vi "Main.vi"(11 "Module Admin":refnum<class "Delacor_lib_QMH_Module Admin.lvclass">) -> ()   [LabVIEW 2023, in "DeviceManager.lvlib"]
doc: "This template is based off of the Queued Message Handler design pattern and the Queued Message Handler project template that ships with LabVIEW.\n\nThe main difference is that the queue is private to this module and communication between modules is performed via Broadcast and Request events.\n\nRequest events are wrapped in public API methods and are handled in the Event Handling Loop (EHL) of this VI. Any module can register for Broadcast events sent by this module. The EHL generates messages based on user interface actions.\n\nThe Message Handling Loop (MHL) processes messages generated by the EHL, or by other messages. The messages are string values, so new messages can be added easily to the Message Cases case structure in the MHL. Each message cluster can also provide an optional value for Message Data, which is a variant that can be converted to whatever message-specific data is required.\n_____\nBased on DQMH Project Template 7.0.0.1280."
uses:
  DeviceManager.lvlib
  <vilib>/Delacor/Delacor QMH/Libraries/Module Admin_class/Delacor_lib_QMH_Module Admin.lvclass
  Module Data--cluster.ctl
  ICLcommuncationData.ctl
  Classes/Communicator/Communicator.lvclass
  OpenWebSocketCommunication (Reply Payload)--cluster.ctl
  SendJSONandAskForReply (Reply Payload)--cluster.ctl
  DiscoverDevices (Reply Payload)--cluster.ctl
  Classes/Mono/Monochromator.lvclass
  Classes/CCD/CCD.lvclass
  Classes/SCD/SCD.lvclass
  <vilib>/Delacor/Delacor QMH/Libraries/Message Queue_class/Delacor_lib_QMH_Message Queue.lvclass/Delacor_lib_QMH_Message Queue.ctl
  Stop Argument--cluster.ctl
  <vilib>/Delacor/Delacor QMH/Libraries/Module Admin_class/Delacor_lib_QMH_Module Admin.lvclass/Delacor_lib_QMH_Module Admin.ctl
  <vilib>/Utility/miscctls.llb/LVPointTypeDef.ctl
  <vilib>/Delacor/Delacor QMH/Libraries/Message Queue_class/Delacor_lib_QMH_Enqueue Message (Single).vi
  <vilib>/Delacor/Delacor QMH/Libraries/Module Admin_class/Delacor_lib_QMH_Get External Launch.vi
  522d4d4e-e2b9-4a0b-813b-57f0bcdbaa64.vi
  <vilib>/GPower/Error/Library/ErrorType.vi
  <vilib>/GPower/Error/Library/SplitAppended.vi
  <vilib>/Utility/error.llb/Trim Whitespace.vi
  <vilib>/GPower/Error/Library/SubVIs/ExplanationToError.vi
  <vilib>/Utility/error.llb/Trim Whitespace One-Sided.vi
  <vilib>/dlg_ctls.llb/Space Constant.vi
  <vilib>/Utility/error.llb/Error Code Database.vi
  <vilib>/GPower/Error/Library/SubVIs/SetStatus.vi
  <vilib>/GPower/Error/Library/AppendErrors.vi
  <vilib>/GPower/Error/Library/Append/AppendSingle.vi
  <vilib>/Delacor/Delacor QMH/Libraries/Message Queue_class/Delacor_lib_QMH_Message Queue.lvclass
  <vilib>/JKI/JKI DotNet System Exec/dotnet_system_exec/dotnet_system_exec.lvclass
  <vilib>/GPower/Error/GPError.lvlib
panel:
  out "ICL output":string caption="StdErr"
  out "StdOut":string
  out "error out":errorcluster
  out "Status":string
  in  "Simulate MHL Error":bool
  in  "Simulate EHL Error":bool
  # "This template is for the DQMH framework. See the block diagram for more information on how to use this template."
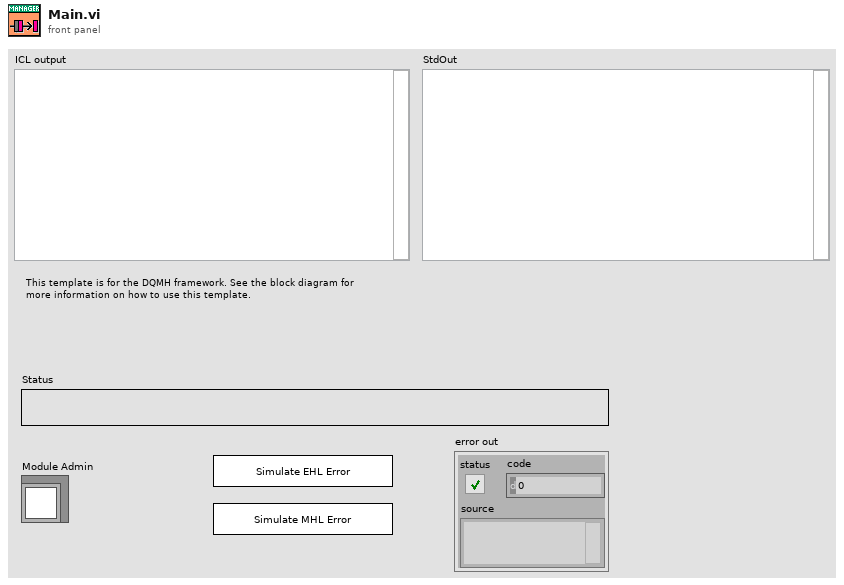
[diagram p1: front panel]
types:
  T1 = cluster{"stdout event":refnum<user-event>, "stderr event":refnum<user-event>, "process_exit event":refnum<user-event>}
  T2 = typedef "DeviceManager.lvlib/Request Events--cluster.ctl" = cluster{"Stop Module":refnum<user-event>, "Show Panel":refnum<user-event>, "Hide Panel":refnum<user-event>, "Get Module Execution Status":refnum<user-event>, "Show Diagram":refnum<user-event>, "StartICL":refnum<user-event>, "OpenWebSocketCommunication":refnum<user-event>, "Private":cluster{"ICLstartNotification":refnum<user-event>}, "ICLshutdown":refnum<user-event>, "SendJSONandAskForReply":refnum<user-event>, "DiscoverDevices":refnum<user-event>}
  T3 = typedef "DeviceManager.lvlib/ICLcommuncationData.ctl" = cluster{"Status":string, "ICL.exe started":bool, "Communicator":refnum<class "Communicator.lvclass">}
  T4 = typedef "DeviceManager.lvlib/Module Data--cluster.ctl" = cluster{"Status":string}
  T5 = typedef "DeviceManager.lvlib/OpenWebSocketCommunication (Reply Payload)--cluster.ctl" = cluster{"Return Headers":variant, "error":errorcluster}
  T6 = typedef "DeviceManager.lvlib/SendJSONandAskForReply (Reply Payload)--cluster.ctl" = cluster{"JSON reply":string, "error":errorcluster}
  T7 = typedef "DeviceManager.lvlib/DiscoverDevices (Reply Payload)--cluster.ctl" = cluster{"Monos":refnum<class "Monochromator.lvclass">[], "CCDs":refnum<class "CCD.lvclass">[], "SCDs":refnum<class "SCD.lvclass">[], "error":errorcluster}
  T8 = enum32{"invalid lock state", "Not Locked", "Locked (No Password)", "Password-protected"}
  T9 = typedef "DeviceManager.lvlib/Stop Argument--cluster.ctl" = cluster{"Origin":string, "Exit via Stop Module Req?":bool, "Wait for Module to stop?":bool}
  T10 = typedef "LVPointTypeDef.ctl" = cluster{"Horizontal":i16, "Vertical":i16}
  T11 = enum32{"Invalid", "Standard", "Closed", "Hidden", "Minimized", "Maximized"}
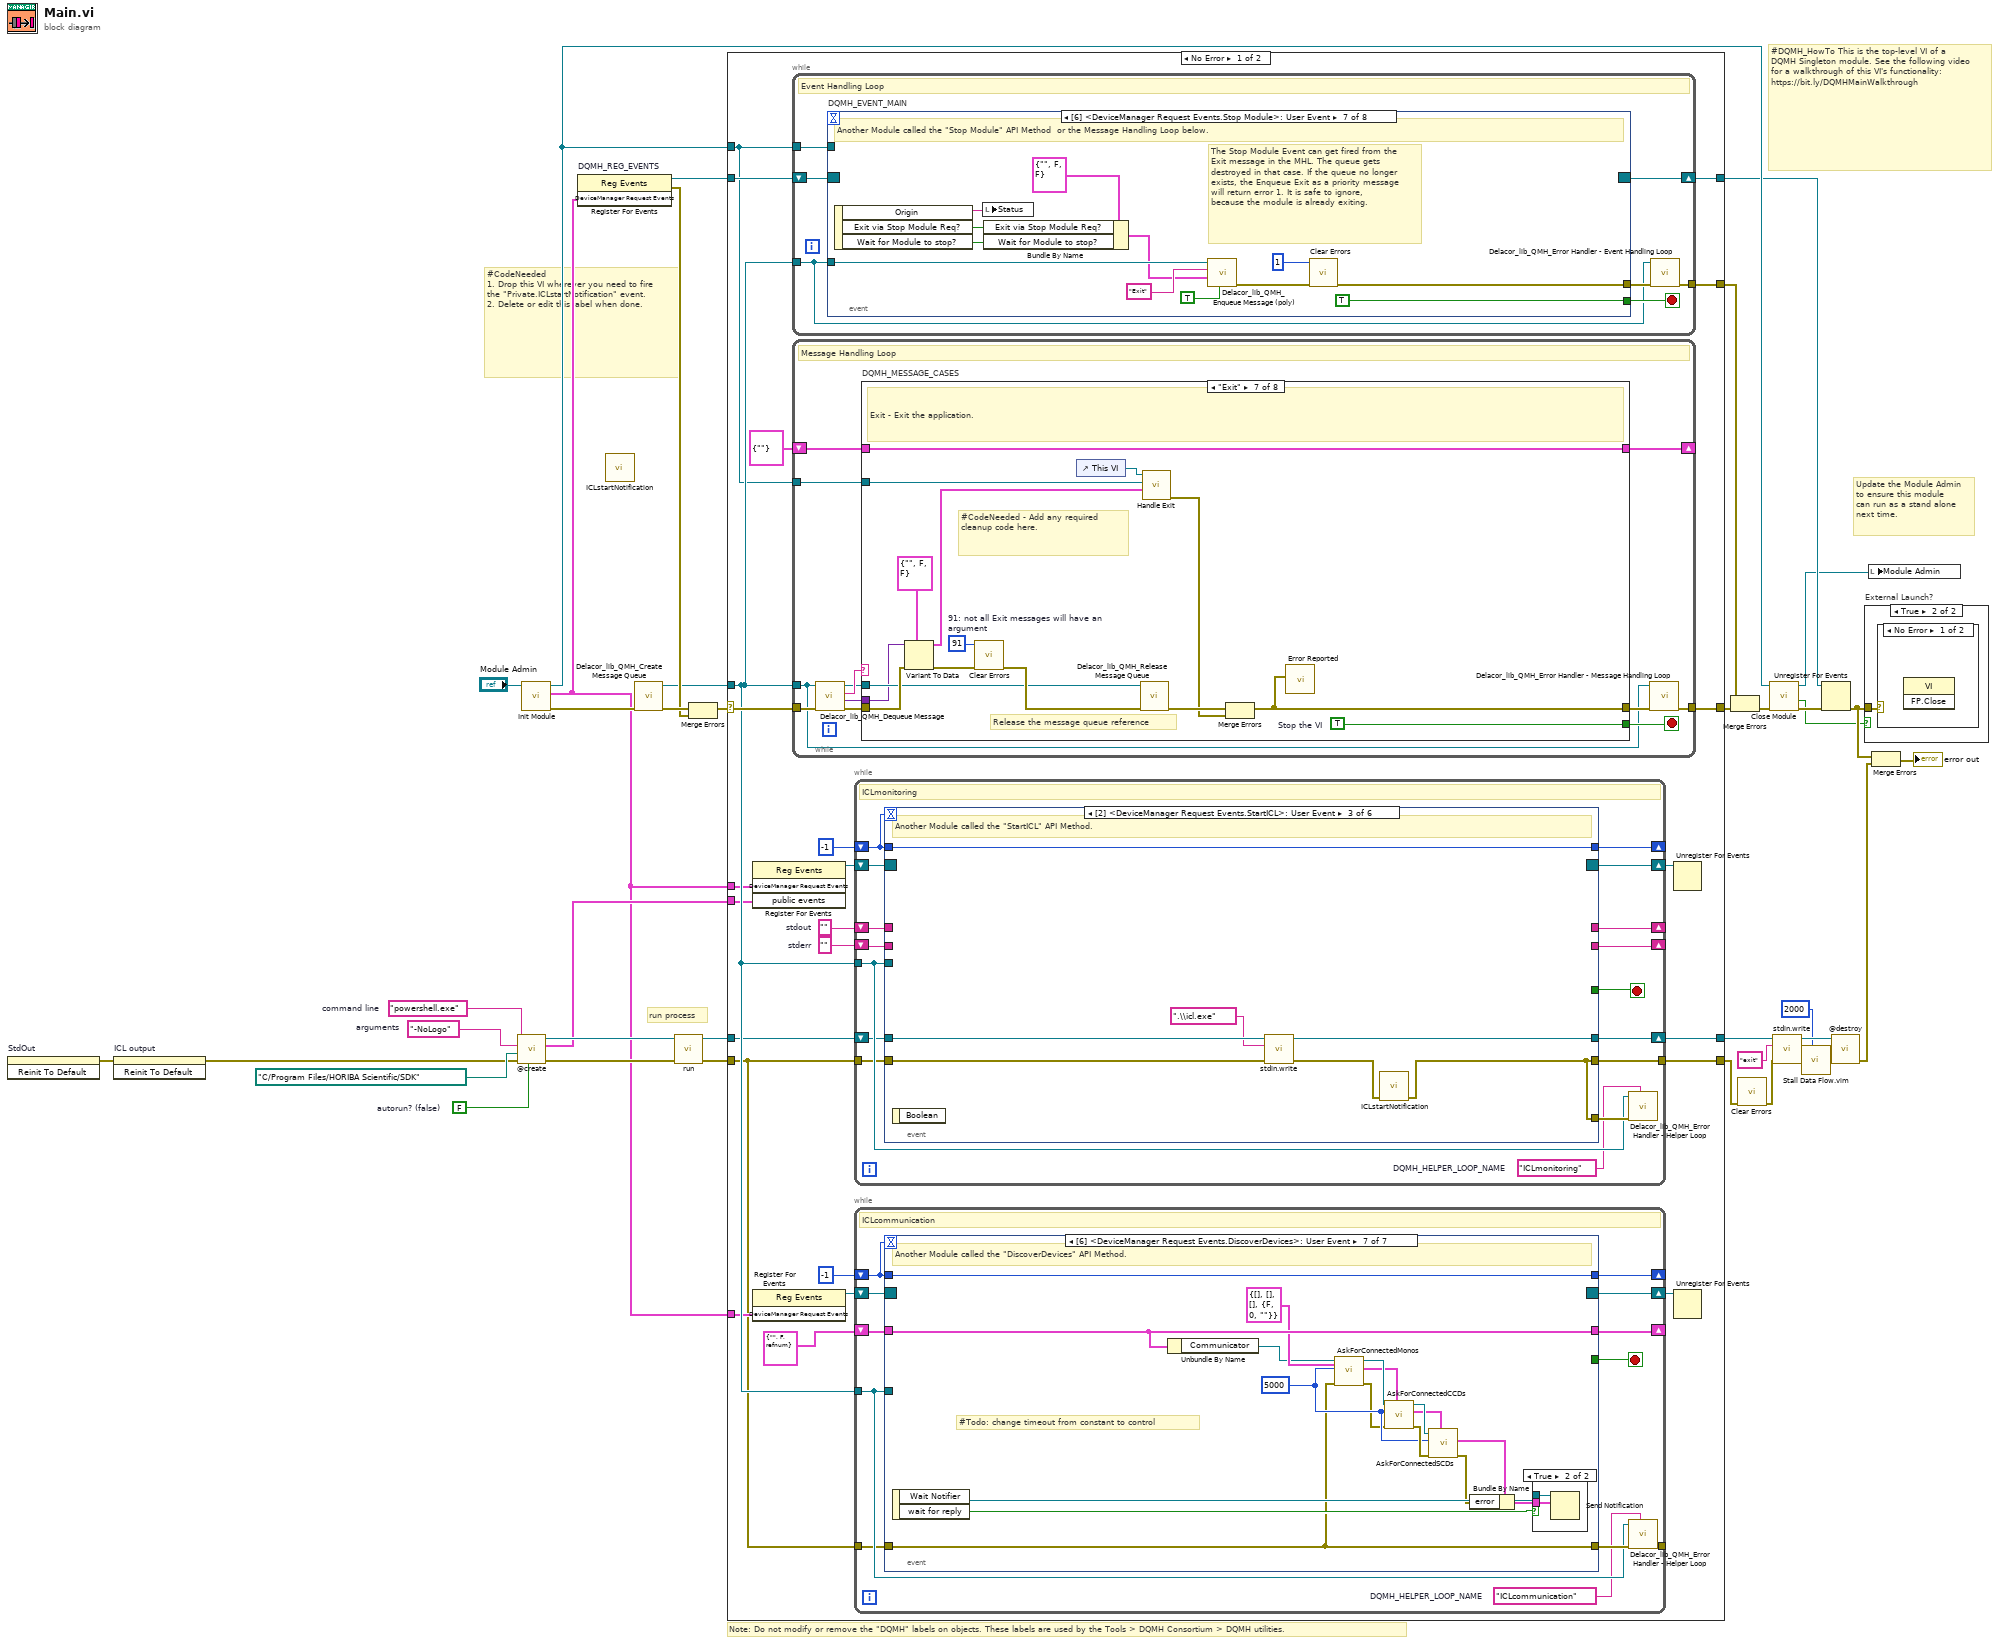
[diagram p0: block diagram]
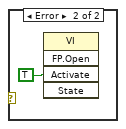
[diagram p3: hidden frame]
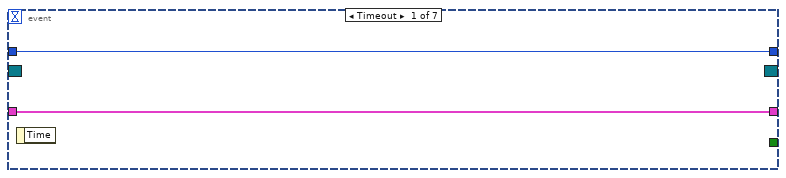
[diagram p4: hidden frame]
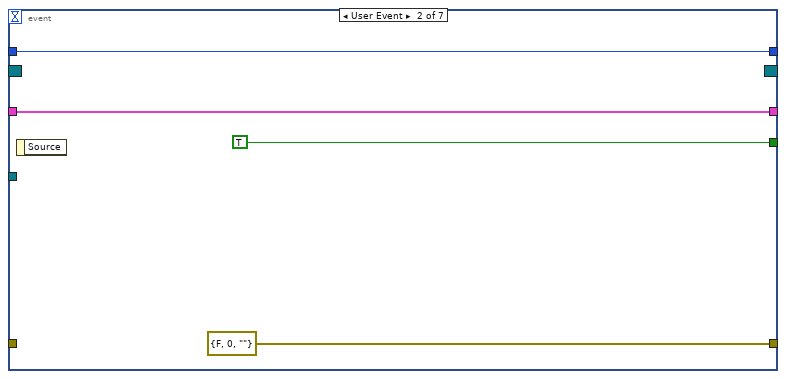
[diagram p5: hidden frame]
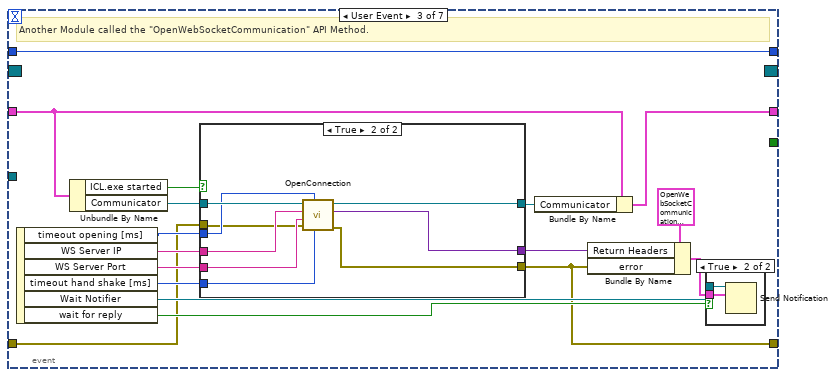
[diagram p6: hidden frame]
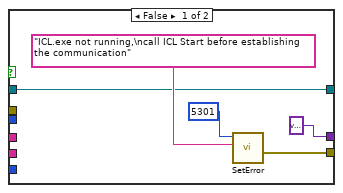
[diagram p7: hidden frame]
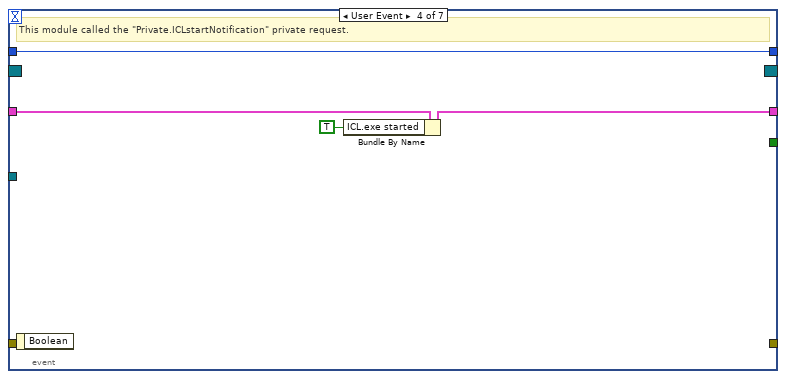
[diagram p9: hidden frame]
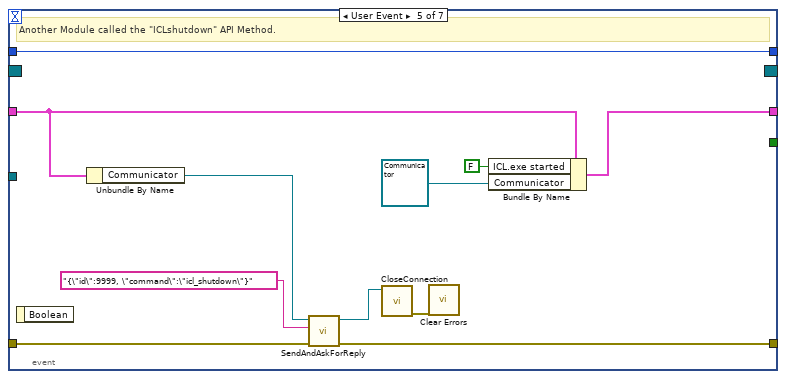
[diagram p10: hidden frame]
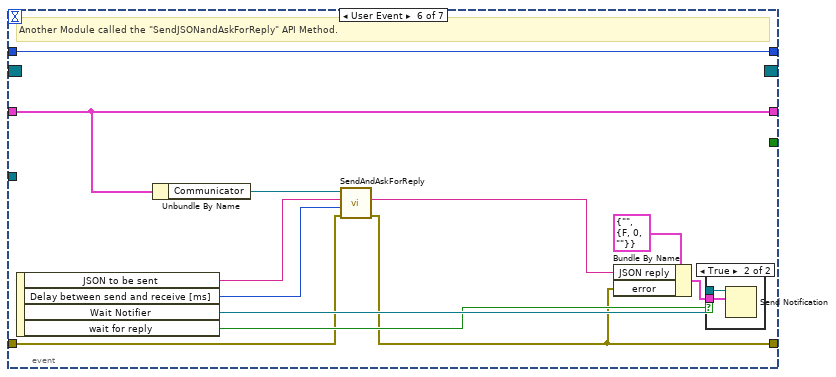
[diagram p11: hidden frame]
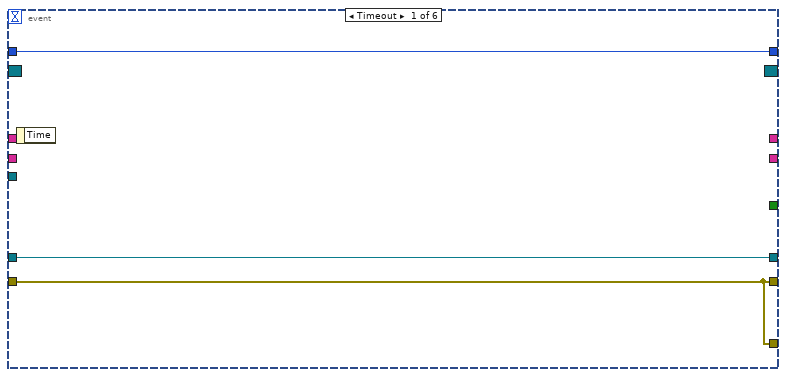
[diagram p14: hidden frame]
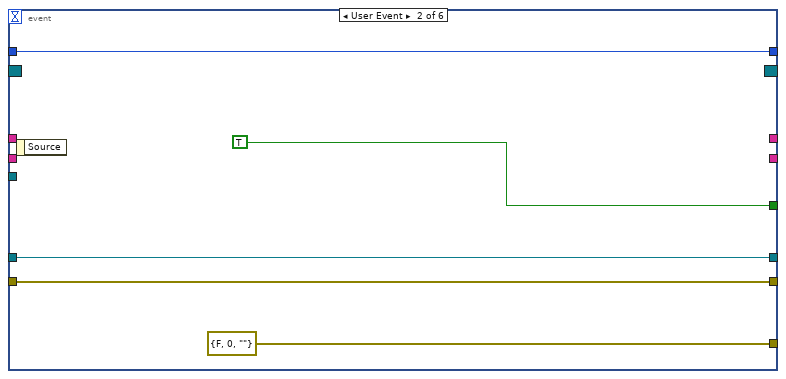
[diagram p15: hidden frame]
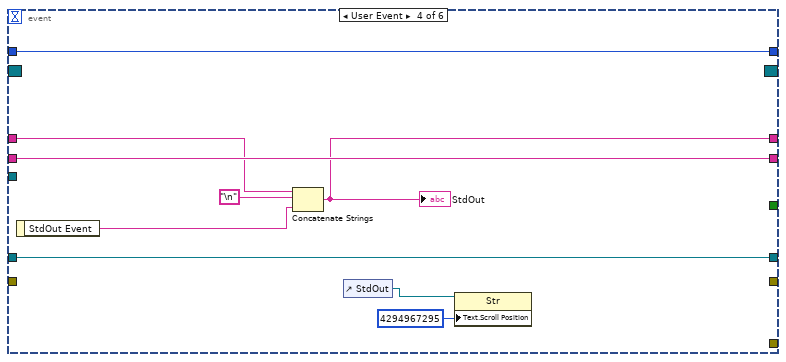
[diagram p16: hidden frame]
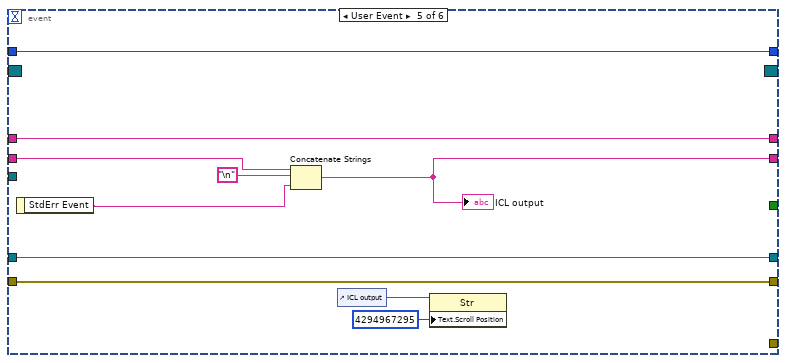
[diagram p17: hidden frame]
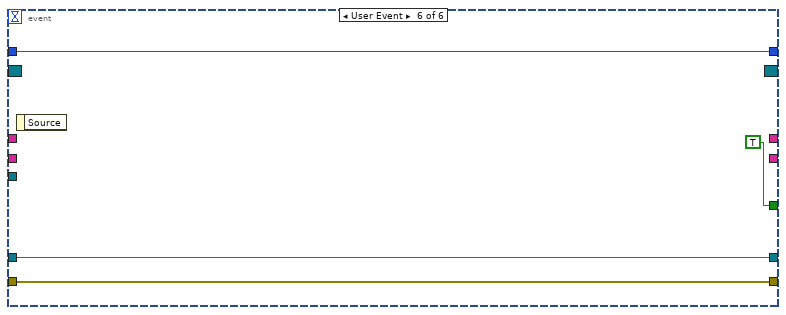
[diagram p18: hidden frame]
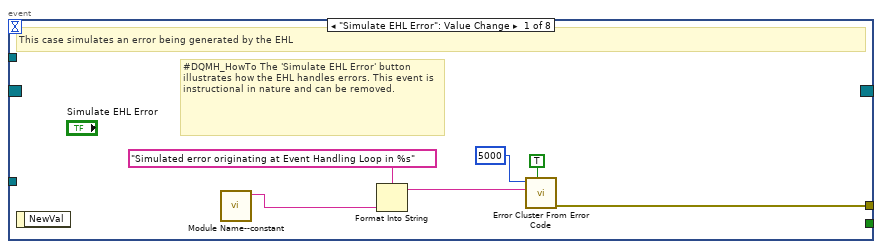
[diagram p19: hidden frame]
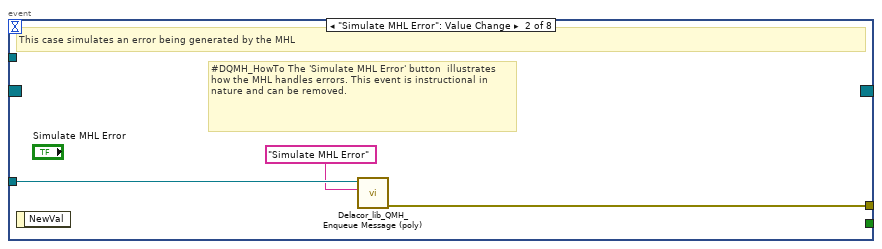
[diagram p20: hidden frame]
diagram:
  w21 = FALSE  # autorun? (false)
  w19 = "-NoLogo"  # arguments
  w18 = "powershell.exe"  # command line
  # "#CodeNeeded\n1. Drop this VI wherever you need to fire the \"Private.ICLstartNotification\" event.\n2. Delete or edit this label when done."
  # "run process"
  # "#DQMH_HowTo This is the top-level VI of a DQMH Singleton module. See the following video for a walkthrough of this VI's functionality: https://bit.ly/DQMHMainWalkthrough"
  # "Note: Do not modify or remove the \"DQMH\" labels on objects. These labels are used by the Tools > DQMH Consortium > DQMH utilities."
  # "Update the Module Admin to ensure this module can run as a stand alone next time."
  n1 = invoke on="StdOut" class="Str" method="Reinit To Default"() -> (error out=w4:errorcluster)  [unwired: 3 in, 2 out]
  n2 = invoke on="ICL output" class="Str" method="Reinit To Default"(error in=w4) -> (error out=w5:errorcluster)  [unwired: 2 in, 2 out]
  n3 = call <vilib>:"@create.vi"("autorun? (false)"=w21, "error in (no error)"=w5, "working directory (c:\\)"=path "C:/Program Files/HORIBA Scientific/SDK" ("working directory"), "arguments (\"\")"=w19, "command line (cmd.exe)"=w18) -> ("error out"=w17:errorcluster, "public events"=w16:T1, "dotnet_system_exec out"=w22:refnum<class "dotnet_system_exec.lvclass">)  [unwired: 4 in]
  n4 = call "Init Module.vi"("Singleton Module Admin in"="Module Admin") -> ("error out"=w37:errorcluster, "DeviceManager Request Events"=w3:T2, "Singleton Module Admin out"=w29:refnum<class "Delacor_lib_QMH_Module Admin.lvclass">)  [unwired: 8 in]
  n5 = register-events "DQMH_REG_EVENTS"(w3) -> (reference out=w27:refnum<event-registration>, error out=w30:errorcluster)  [unwired: 2 in]
  n6 = call "ICLstartNotification.vi"() -> ()  [unwired: 11 in, 1 out]
  n7 = call <vilib>:"Delacor_lib_QMH_Create Message Queue.vi"("error in"=w37) -> ("error out"=w32:errorcluster, "Message Queue"=w26:refnum<class "Delacor_lib_QMH_Message Queue.lvclass">)  [unwired: 9 in]
  n8 = call <vilib>:"run.vi"("error in (no error)"=w17, "dotnet_system_exec in"=w22) -> ("error out"=w15:errorcluster, "dotnet_system_exec out"=w14:refnum<class "dotnet_system_exec.lvclass">)  [unwired: 8 in]
  n9 = Merge Errors(w32, w30) -> (w31:errorcluster)
  n10 = case shown="No Error" w31 {
    selector: w31 -> [w60 w370]
    tunnel: [w62 w369] -> w38
    tunnel: [w59 w368] -> w28
    tunnel: w27 -> [w57 w368]
    tunnel: w26 -> [w56 w363]
    tunnel: [w61 _] -> w35
    tunnel: w29 -> [w55 w364]
    tunnel: w3 -> [w54 _]
    tunnel: w16 -> [w50 _]
    tunnel: w15 -> [w39 w362]
    tunnel: w14 -> [w49 w361]
    tunnel: [w48 w361] -> w12
    tunnel: [w47 w362] -> w11
    tunnel: w3 -> [w44 _]
    frame No Error {
      w45 = ""  # stderr
      w46 = ""  # stdout
      n11 = register-events ("DQMH_HELPER_REGFOREVENTS")(w54, w50) -> (reference out=w52:refnum<event-registration>)  [unwired: 2 in, 1 out]
      n12 = register-events ("DQMH_HELPER_REGFOREVENTS")(w44) -> (reference out=w42:refnum<event-registration>)  [unwired: 2 in, 1 out]
      n13 = while {
        tunnel: w56 -> [w216]
        shift-right: [w219] -> w59
        shift-left: w57 -> [w220]
        tunnel: [w221] -> w61
        tunnel: w55 -> [w217]
        stop <- w218 stop-if-true
        # "Event Handling Loop"
        n14 = event "DQMH_EVENT_MAIN" shown="[6] <DeviceManager Request Events.Stop Module>: User Event" {
          selector: w220 -> [_ _ _ _ _ _ _ _]
          dyn-events: [_ _ _ _ _ _ _ _] -> w219
          timeout: _ -> [_ _ _ _ _ _ _ _]
          tunnel: [_ _ _ _ _ _ TRUE ("Discard?") _] -> w218
          tunnel: w216 -> [_ w230 _ _ _ _ w254 w261]
          tunnel: [w228 w231 _ _ w237 _ w257 w263] -> w222
          tunnel: w217 -> [_ _ _ _ _ _ _ w260]
          event "Simulate EHL Error": Value Change {
            # "#DQMH_HowTo The 'Simulate EHL Error' button  illustrates how the EHL handles errors. This event is instructional in nature and can be removed."
            # "This case simulates an error being generated by the EHL"
            n15 = event-data() -> ()  [unwired: 1 in, 1 out]
            n16 = call "Module Name--constant.vi"() -> ("Module Name"=w225:string)  [unwired: 11 in]
            n17 = Format Into String(format string="Simulated error originating at Event Handling Loop in %s", w225) -> (resulting string=w226:string)  [unwired: 2 in, 1 out]
            n18 = call <vilib>:"Error Cluster From Error Code.vi"("show call chain? (False)"=TRUE, "error message (\"\")"=w226, "error code (0)"=5000) -> ("error out"=w228:errorcluster)  [unwired: 6 in]
          }
          event "Simulate MHL Error": Value Change {
            # "#DQMH_HowTo The 'Simulate MHL Error' button  illustrates how the MHL handles errors. This event is instructional in nature and can be removed."
            # "This case simulates an error being generated by the MHL"
            n19 = event-data() -> ()  [unwired: 1 in, 1 out]
            n20 = call-poly <vilib>:"Delacor_lib_QMH_Enqueue Message (poly).vi"("Message"="Simulate MHL Error", "Message Queue in"=w230) -> ("error out"=w231:errorcluster)  [unwired: 8 in, 1 out]
          }
          event User Event {
            # "Show the panel of this VI, and send a status updated message to let listeners know."
            # "Another Module called the \"Show Panel\" API Method."
            n21 = event-data() -> ()  [unwired: 1 in, 1 out]
            n22 = control-ref of="This VI"() -> (w233:refnum<vi>)
            n23 = call "Open VI Panel.vi"("VI"=w233) -> ()  [unwired: 10 in, 1 out]
            n24 = call "Status Updated.vi"("Status"="Panel shown." ("format string")) -> ()  [unwired: 10 in, 1 out]
          }
          event User Event {
            # "Hide the panel of this VI, and send a status updated message to let listeners know."
            # "Another Module called the \"Hide Panel\" API Method."
            n25 = event-data() -> ()  [unwired: 1 in, 1 out]
            n26 = control-ref of="This VI"() -> (w235:refnum<vi>)
            n27 = call "Hide VI Panel.vi"("VI"=w235) -> ()  [unwired: 10 in, 1 out]
            n28 = call "Status Updated.vi"("Status"="Panel hidden." ("format string")) -> ()  [unwired: 10 in, 1 out]
          }
          event User Event {
            # "Another Module called the \"Get Module Execution Status\" API Method."
            n29 = event-data() -> ()  [unwired: 1 in, 1 out]
            n30 = call "Update Module Execution Status.vi"("Running?"=TRUE) -> ("error out"=w237:errorcluster)  [unwired: 10 in]
          }
          event User Event {
            # "Another Module called the \"Show Diagram\" API Method. This event is used for debugging."
            n31 = event-data() -> ()  [unwired: 1 in, 1 out]
            n32 = disable-structure shown="RUN_TIME_ENGINE==False" {
              frame condition #0 (active) {
                # "functionality not available in exe"
                n33 = invoke class="VI" method="Lock State.Get"() -> (error out=w243:errorcluster, "Get Lock State"=w242:T8, "pwd in cache"=w239:bool)  [unwired: 4 in, 1 out]
                n34 = Equal?(x=T8."Password-protected", y=w242) -> (x = y?=w240:bool)
                n35 = Compound Arithmetic op=AND(w240, invert w239) -> (w238:bool)
                n36 = case shown="False" w238 {
                  tunnel: w243 -> [w246 _]
                  frame False {
                    n37 = property class="VI"(error in=w246, "BDWin.Open"=TRUE ("Block Diagram Window:Open")) -> ()  [unwired: 1 in, 2 out]
                    n38 = call "Status Updated.vi"("Status"="Block Diagram shown." ("format string")) -> ()  [unwired: 10 in, 1 out]
                  }
                  frame True {
                    # "Password-protected VI, and the password is not in the cache. Do not show the diagram."
                  }
                }
              }
              frame condition #1 {
              }
            }
          }
          event User Event {
            # "The Stop Module Event can get fired from the Exit message in the MHL. The queue gets destroyed in that case. If the queue no longer exists, the Enqueue Exit as a priority message will return error 1. It is safe to ignore, because the module is already exiting."
            # "Another Module called the \"Stop Module\" API Method  or the Message Handling Loop below."
            n39 = event-data() -> ("Origin"=w253:string, "Exit via Stop Module Req?"=w249:bool, "Wait for Module to stop?"=w248:bool)  [unwired: 1 in]
            n40 = local write "Status"(w253) -> ()
            n41 = Bundle By Name(cluster=T9 {"Origin"="", "Exit via Stop Module Req?"=FALSE, "Wait for Module to stop?"=FALSE} ("Stop Argument"), "Exit via Stop Module Req?"=w249, "Wait for Module to stop?"=w248) -> (w247:T9)
            n42 = call-poly <vilib>:"Delacor_lib_QMH_Enqueue Message (poly).vi"("Priority Message? (F)"=TRUE, "Message Data"=w247, "Message"="Exit", "Message Queue in"=w254) -> ("error out"=w258:errorcluster)  [unwired: 6 in, 1 out]
            n43 = call <vilib>:"Clear Errors.vi"("error in (no error)"=w258, "specific error code to clear (0: all)"=1) -> ("error out"=w257:errorcluster)  [unwired: 4 in, 1 out]
          }
          event Panel Close? {
            w262 = TRUE  # Discard the event, the MHL is responsible for closing and stopping this VI.
            # "Hide the panel or send the 'Exit' message if the user clicks the 'X' on the module main VI panel."
            n44 = event-data() -> ()  [unwired: 1 in, 1 out]
            n45 = property class="Module Admin"(reference=w260) -> ("Accessors:External Launch"=w259:bool)  [unwired: 1 in, 2 out]
            n46 = case shown="True" w259 {
              tunnel: w261 -> [_ w269]
              tunnel: [_ w270] -> w263
              frame True {
                # "If externally launched, clicking the 'X' hides the panel, but doesn't close it."
                n47 = control-ref of="This VI"() -> (w266:refnum<vi>)
                n48 = call "Hide VI Panel.vi"("VI"=w266) -> ("error out"=w264:errorcluster)  [unwired: 10 in]
                n49 = call "Status Updated.vi"("error in"=w264, "Status"="Panel hidden." ("format string")) -> ()  [unwired: 9 in, 1 out]
              }
              frame False {
                # "If run as a stand-alone VI, clicking the panel 'X' stops the VI."
                n50 = call-poly <vilib>:"Delacor_lib_QMH_Enqueue Message (poly).vi"("Priority Message? (F)"=TRUE, "Message"="Exit", "Message Queue in"=w269) -> ("error out"=w270:errorcluster)  [unwired: 7 in, 1 out]
              }
            }
            n51 = event-data("Discard?"=w262) -> ()  [unwired: 1 in, 1 out]
          }
        }
        n52 = call-dynamic "Delacor_lib_QMH_Error Handler - Event Handling Loop.vi"("error in"=w222, "Message Queue in"=w216) -> ("dup error in"=w221:errorcluster)  [unwired: 8 in, 1 out]
      }
      n53 = while {
        tunnel: w56 -> [w271]
        shift-right: [w277] -> _
        shift-left: T4 {"Status"=""} ("Data Cluster") -> [w278]
        tunnel: w60 -> [w281]
        tunnel: [w279] -> w62
        tunnel: w55 -> [w272]
        stop <- w276 stop-if-true
        # "Message Handling Loop"
        n54 = call-dynamic "Delacor_lib_QMH_Dequeue Message.vi"("error in"=w281, "Message Queue in"=w271) -> ("error out"=w280:errorcluster, "Message Data"=w274:variant, "Message"=w275:string, "Message Queue out"=w273:refnum<class "Delacor_lib_QMH_Message Queue.lvclass">)  [unwired: 6 in]
        n55 = case "DQMH_MESSAGE_CASES" shown="\"Exit\"" w275 {
          selector: w275 -> [_ _ _ _ _ _ _ w356]
          tunnel: w273 -> [_ _ _ _ _ w322 w344 _]
          tunnel: w280 -> [w300 w304 w307 w309 w318 w329 w350 w359]
          tunnel: [w298 w304 w306 w309 w317 w325 w345 w360] -> w282
          tunnel: w278 -> [w289 w303 w305 w308 w315 w324 w343 w357]
          tunnel: [w288 w303 w305 w308 w315 w324 w343 w357] -> w277
          tunnel: [_ _ _ _ _ _ w342 _] -> w276
          tunnel: w274 -> [_ _ _ _ _ w323 w341 _]
          tunnel: w272 -> [w290 _ _ _ _ w321 w336 _]
          frame "Initialize" {
            w284 = "Initial Message" ("Initial Message")
            # "#CodeNeeded - Initialize the appearance of the front panel."
            # "#CodeNeeded - Initialize your state data here."
            # "Initialize - Any operation that needs to be done before the module can receive messages. Synchronize Caller Events.vi will inform Start Module.vi that the module has launched and is ready to receive messages. Module Did Init.vi will broadcast that the module initialized."
            n56 = call "Synchronize Caller Events.vi"("error in"=w300, "Singleton Module Admin in"=w290) -> ("error out"=w299:errorcluster, "Singleton Module Admin out"=w285:refnum<class "Delacor_lib_QMH_Module Admin.lvclass">)  [unwired: 8 in]
            n57 = property class="Module Admin"(reference=w285) -> ("Accessors:External Launch"=w294:bool)  [unwired: 1 in, 2 out]
            n58 = Select(t=T11."Hidden" ("State"), s=w294, f=T11."Standard" ("State")) -> (s? t:f=w291:T11)
            n59 = call "Module Name--constant.vi"() -> ("Module Name"=w297:string)  [unwired: 11 in]
            n60 = property class="VI"("Front Panel.Title"=w297) -> (reference out=w296:refnum<vi>, error out=w302:errorcluster)  [unwired: 2 in]
            n61 = call "Module Name--constant.vi"() -> ("Module Name"=w286:string)  [unwired: 11 in]
            n62 = invoke class="VI" method="FP.Open"(reference=w296, error in=w302, "State"=w291) -> (reference out=w295:refnum<vi>, error out=w301:errorcluster)  [unwired: 2 in, 3 out]
            n63 = Bundle By Name(cluster=w289, "Status"=w284) -> (w288:T4)
            n64 = call "Module Did Init.vi"("error in"=w299, "Initialized?"=TRUE, "Origin"=w286) -> ("error out"=w298:errorcluster)  [unwired: 8 in]
            n65 = invoke class="VI" method="FP.Center"(reference=w295, error in=w301) -> ()  [unwired: 1 in, 3 out]
            n66 = property on="Pane" class="Pane"("Origin"=T10 {"Horizontal"=0, "Vertical"=0}) -> ()  [unwired: 2 in, 2 out]
            "Status" <- w284
          }
          frame "---Module Specific---" {
            # "Separator -- The following cases handle messages specific to this Module."
          }
          frame "---Copy This Frame---" {
            # "Duplicate this frame when creating new messages.  Change this comment in the duplicated frame to describe this message."
            n67 = Merge Errors(w307) -> (w306:errorcluster)
          }
          frame "---Exit and Error Handling---" {
            # "Separator - The following cases handle errors and exit messages."
          }
          frame "Simulate MHL Error" {
            # "#DQMH_HowTo The 'Simulate MHL Error' button  illustrates how the MHL handles errors. This event is instructional in nature and can be removed."
            # "Simulate an error occurring at the MHL"
            n68 = call "Module Name--constant.vi"() -> ("Module Name"=w311:string)  [unwired: 11 in]
            n69 = Format Into String(format string="Simulated error originating at Message Handling Loop in %s", w311) -> (resulting string=w312:string)  [unwired: 2 in, 1 out]
            n70 = call <vilib>:"Error Cluster From Error Code.vi"("show call chain? (False)"=TRUE, "error message (\"\")"=w312, "error code (0)"=5001) -> ("error out"=w316:errorcluster)  [unwired: 6 in]
            n71 = Merge Errors(w318, w316) -> (w317:errorcluster)
          }
          frame "Error" {
            # "#CodeRecommended - If the module is running in standalone mode (External Launch = FALSE), this code will pop up an error dialog and call the 'Exit' message if an error occurs. Add more fine-grained error management here."
            # "Error - Check the error message data and respond accordingly. This message is sent by the \"Error Handler\" VIs at the end of each loop in this application."
            n72 = property class="Module Admin"(reference=w321) -> ("Accessors:External Launch"=w320:bool)  [unwired: 1 in, 2 out]
            n73 = Variant To Data(error in=w329, type=errorcluster {"status"=FALSE, "code"=0, "source"=""} ("error constant"), Variant=w323) -> (data=w319:errorcluster, error out=w327:errorcluster)
            n74 = local write "error out"(w319) -> ()
            n75 = call "Error Reported.vi"("Error"=w319) -> ()  [unwired: 10 in, 1 out]
            n76 = case shown="False" w320 {
              tunnel: [w334 _] -> w326
              tunnel: w322 -> [w332 _]
              tunnel: w319 -> [w333 _]
              frame False {
                n77 = disable-structure shown="Default" {
                  disable-tunnel: w333 -> [w335 _]
                  frame condition #0 (active) {
                    # "If the module is running standalone, then pop up an error dialog and call the \"Exit\" message."
                    n78 = call <vilib>:"Simple Error Handler.vi"("error in (no error)"=w335) -> ()  [unwired: 4 in, 5 out]
                  }
                  frame condition #1 {
                    # "To prevent the Simple Error Handler VI from being loaded (e.g. when deploying to a Real-Time target), add the Conditional Disable Symbol \"DQMH_Disable_SEH\" to your project and set it to TRUE."
                  }
                }
                n79 = call-poly <vilib>:"Delacor_lib_QMH_Enqueue Message (poly).vi"("Priority Message? (F)"=TRUE, "Message"="Exit", "Message Queue in"=w332) -> ("error out"=w334:errorcluster)  [unwired: 7 in, 1 out]
              }
              frame True {
                # "If the module was launched externally, calling the Error Reported broadcast VI is the only action performed by the \"Error\" message. The module's caller can then process the error appropriately."
              }
            }
            n80 = Merge Errors(w327, w326) -> (w325:errorcluster)
          }
          frame "Exit" {
            w340 = 91  # 91: not all Exit messages will have an argument
            w342 = TRUE  # Stop the VI
            # "Release the message queue reference"
            # "#CodeNeeded - Add any required cleanup code here."
            # "Exit - Exit the application."
            n81 = Variant To Data(error in=w350, type=T9 {"Origin"="", "Exit via Stop Module Req?"=FALSE, "Wait for Module to stop?"=FALSE} ("Stop Argument"), Variant=w341) -> (data=w338:T9, error out=w347:errorcluster)
            n82 = call <vilib>:"Clear Errors.vi"("error in (no error)"=w347, "specific error code to clear (0: all)"=w340) -> ("error out"=w349:errorcluster)  [unwired: 4 in, 1 out]
            n83 = control-ref of="This VI"() -> (w337:refnum<vi>)
            n84 = call-dynamic "Delacor_lib_QMH_Release Message Queue.vi"("error in"=w349, "Message Queue"=w344) -> ("error out"=w348:errorcluster)  [unwired: 9 in]
            n85 = call "Handle Exit.vi"("Stop Argument"=w338, "Admin in"=w336, "VI reference"=w337) -> ("error out"=w346:errorcluster)  [unwired: 7 in, 1 out]
            n86 = Merge Errors(w348, w346) -> (w345:errorcluster)
            n87 = call "Error Reported.vi"("Error"=w345) -> ()  [unwired: 10 in, 1 out]
          }
          frame Default {
            # "'Default' case only runs if there is a message that isn't defined in any of the other cases.  Output a programming error."
            n88 = call "Module Name--constant.vi"() -> ("Module Name"=w355:string)  [unwired: 11 in]
            n89 = Format Into String(format string="The invalid message string \"%s\" was received in the Message Handling Loop for module \"%s\".", w356, w355) -> (resulting string=w351:string)  [unwired: 2 in, 1 out]
            n90 = call <vilib>:"Error Cluster From Error Code.vi"("show call chain? (False)"=TRUE, "error message (\"\")"=w351, "error code (0)"=1) -> ("error out"=w358:errorcluster)  [unwired: 6 in]
            n91 = Merge Errors(w359, w358) -> (w360:errorcluster)
          }
        }
        n92 = call-dynamic "Delacor_lib_QMH_Error Handler - Message Handling Loop.vi"("error in"=w282, "Message Queue in"=w271) -> ("dup error in"=w279:errorcluster)  [unwired: 8 in, 1 out]
      }
      n93 = while "DQMH_HELPER_LOOP" {
        shift-right: [w177] -> _
        shift-left: -1 -> [w176]
        shift-right: [w174] -> w53
        shift-left: w52 -> [w175]
        tunnel: w56 -> [w171]
        tunnel: w39 -> [w169]
        shift-right: [w166] -> w48
        shift-left: w49 -> [w168]
        tunnel: [w167] -> w47
        shift-right: [w162] -> _
        shift-left: w46 -> [w163]
        shift-right: [w165] -> _
        shift-left: w45 -> [w164]
        stop <- w173 stop-if-true
        w170 = "ICLmonitoring"  # DQMH_HELPER_LOOP_NAME
        # "ICLmonitoring"
        n94 = event "DQMH_HELPER_EVENT_STRUCTURE" shown="[2] <DeviceManager Request Events.StartICL>: User Event" {
          selector: w175 -> [_ _ _ _ _ _]
          dyn-events: [_ _ _ _ _ _] -> w174
          timeout: w176 -> [_ _ _ _ _ _]
          tunnel: w176 -> [w180 w185 w192 w201 w211 w215]
          tunnel: [w180 w185 w192 w201 w211 w215] -> w177
          tunnel: [_ TRUE _ _ _ TRUE] -> w173
          tunnel: [w178 errorcluster {"status"=FALSE, "code"=0, "source"=""} ("error constant") w186 _ _ _] -> w172
          tunnel: w171 -> [_ _ _ _ _ _]
          tunnel: w169 -> [w178 w181 w189 _ w202 w212]
          tunnel: w168 -> [w179 w182 w190 w200 w210 w214]
          tunnel: [w178 w181 w186 _ w202 w212] -> w167
          tunnel: [w179 w182 w191 w200 w210 w214] -> w166
          tunnel: [_ _ _ w199 w205 _] -> w165
          tunnel: w164 -> [_ _ _ w199 w208 _]
          tunnel: w163 -> [_ _ _ w197 w206 _]
          tunnel: [_ _ _ w195 w206 _] -> w162
          event Timeout {
            n95 = event-data() -> ()  [unwired: 1 in, 1 out]
          }
          event User Event {
            n96 = event-data() -> ()  [unwired: 1 in, 1 out]
          }
          event User Event {
            # "Another Module called the \"StartICL\" API Method."
            n97 = event-data() -> ()  [unwired: 1 in, 1 out]
            n98 = call-dynamic "stdin.write.vi"("error in (no error)"=w189, "stdin"=".\\icl.exe", "dotnet_system_exec in"=w190) -> ("error out"=w187:errorcluster, "dotnet_system_exec out"=w191:refnum<class "dotnet_system_exec.lvclass">)  [unwired: 7 in]
            n99 = call "ICLstartNotification.vi"("error in"=w187) -> ("error out"=w186:errorcluster)  [unwired: 10 in]
          }
          event User Event {
            n100 = event-data() -> ("StdOut Event"=w196:string)  [unwired: 1 in]
            n101 = Concatenate Strings(w197, "\n", w196) -> (w195:string)
            "StdOut" <- w195
            n102 = control-ref of="StdOut"() -> (w194:refnum<vi>)
            n103 = property on="Property Node" class="Str"(reference=w194, "Text.Scroll Position"=u32 4294967295) -> ()  [unwired: 1 in, 2 out]
          }
          event User Event {
            n104 = event-data() -> ("StdErr Event"=w207:string)  [unwired: 1 in]
            n105 = Concatenate Strings(w208, "\n", w207) -> (w205:string)
            "ICL output" <- w205
            n106 = control-ref of="ICL output"() -> (w203:refnum<vi>)
            n107 = property on="Property Node" class="Str"(reference=w203, "Text.Scroll Position"=u32 4294967295) -> ()  [unwired: 1 in, 2 out]
          }
          event User Event {
            n108 = event-data() -> ()  [unwired: 1 in, 1 out]
          }
        }
        n109 = call-dynamic "Delacor_lib_QMH_Error Handler - Helper Loop.vi"("Error Debug"=w170, "error in"=w172, "Message Queue in"=w171) -> ()  [unwired: 7 in, 2 out]
      }
      n110 = while "DQMH_HELPER_LOOP" {
        shift-right: [w74] -> _
        shift-left: -1 -> [w73]
        shift-right: [w71] -> w43
        shift-left: w42 -> [w72]
        tunnel: w56 -> [w68]
        shift-right: [w65] -> _
        shift-left: T3 {"Status"="", "ICL.exe started"=FALSE, "Communicator"=refnum} ("Data Cluster") -> [w66]
        tunnel: [w64] -> _
        tunnel: w39 -> [w63]
        stop <- w70 stop-if-true
        w67 = "ICLcommunication"  # DQMH_HELPER_LOOP_NAME
        # "ICLcommunication"
        n111 = event "DQMH_HELPER_EVENT_STRUCTURE" shown="[6] <DeviceManager Request Events.DiscoverDevices>: User Event" {
          selector: w72 -> [_ _ _ _ _ _ _]
          dyn-events: [_ _ _ _ _ _ _] -> w71
          timeout: w73 -> [_ _ _ _ _ _ _]
          tunnel: w73 -> [w76 w80 w97 w117 w128 w140 w159]
          tunnel: [w76 w80 w97 w117 w128 w140 w159] -> w74
          tunnel: [_ TRUE _ _ _ _ _] -> w70
          tunnel: [_ errorcluster {"status"=FALSE, "code"=0, "source"=""} ("error constant") w82 _ w124 w129 w144] -> w69
          tunnel: w68 -> [_ _ _ _ _ _ _]
          tunnel: w66 -> [w75 w77 w84 w116 w120 w135 w155]
          tunnel: [w75 w77 w85 w115 w121 w135 w155] -> w65
          tunnel: w63 -> [_ _ w81 _ w125 w132 w144]
          event Timeout {
            n112 = event-data() -> ()  [unwired: 1 in, 1 out]
          }
          event User Event {
            n113 = event-data() -> ()  [unwired: 1 in, 1 out]
          }
          event User Event {
            # "Another Module called the \"OpenWebSocketCommunication\" API Method."
            n114 = event-data() -> ("timeout opening [ms]"=w86:i32, "WS Server IP"=w88:string, "WS Server Port"=w89:string, "timeout hand shake [ms]"=w87:i32, "Wait Notifier"=w96:refnum<notifier>, "wait for reply"=w95:bool)  [unwired: 1 in]
            n115 = Unbundle By Name(w84) -> ("ICL.exe started"=w92:bool, "Communicator"=w90:refnum<class "Communicator.lvclass">)
            n116 = case shown="True" w92 {
              tunnel: [w100 w106] -> w82
              tunnel: [variant ("Return Headers") w105] -> w91
              tunnel: w90 -> [w98 w111]
              tunnel: w89 -> [_ w110]
              tunnel: w88 -> [_ w109]
              tunnel: w87 -> [_ w108]
              tunnel: w86 -> [_ w107]
              tunnel: [w98 w104] -> w83
              tunnel: w81 -> [_ w103]
              frame False {
                n117 = call <vilib>:"SetError.vi"("Error description"="ICL.exe not running,\ncall ICL Start before establishing the communication", "Error code"=5301) -> ("Error out"=w100:errorcluster)  [unwired: 9 in]
              }
              frame True {
                n118 = call-dynamic "OpenConnection.vi"("timeout hand shake [ms]"=w108, "timeout opening [ms]"=w107, "error in (no error)"=w103, "WS Server Port"=w110, "WS Server IP"=w109, "Communicator in"=w111) -> ("error out"=w106:errorcluster, "Return Headers"=w105:variant, "Communicator out"=w104:refnum<class "Communicator.lvclass">)  [unwired: 3 in]
              }
            }
            n119 = Bundle By Name(cluster=w84, "Communicator"=w83) -> (w85:T3)
            n120 = Bundle By Name(cluster=T5 {"Return Headers"=variant, "error"={"status"=FALSE, "code"=0, "source"=""}} ("OpenWebSocketCommunication (Reply Payload)"), "Return Headers"=w91, "error"=w82) -> (w94:T5)
            n121 = case "DQMH_FIRE_NOTIFIER" shown="True" w95 {
              tunnel: w96 -> [_ w113]
              tunnel: w94 -> [_ w112]
              frame False {
              }
              frame True {
                n122 = Send Notification(notification=w112, notifier=w113) -> ()  [unwired: 1 in, 2 out]
              }
            }
          }
          event User Event {
            # "This module called the \"Private.ICLstartNotification\" private request."
            n123 = event-data() -> ()  [unwired: 1 in, 1 out]
            n124 = Bundle By Name(cluster=w116, "ICL.exe started"=TRUE) -> (w115:T3)
          }
          event User Event {
            # "Another Module called the \"ICLshutdown\" API Method."
            n125 = event-data() -> ()  [unwired: 1 in, 1 out]
            n126 = Unbundle By Name(w120) -> ("Communicator"=w127:refnum<class "Communicator.lvclass">)
            n127 = call-dynamic "SendAndAskForReply.vi"("error in (no error)"=w125, "String to be sent"="{\"id\":9999, \"command\":\"icl_shutdown\"}", "Communicator in"=w127) -> ("error out"=w124:errorcluster, "Communicator out"=w123:refnum<class "Communicator.lvclass">)  [unwired: 6 in, 1 out]
            n128 = call-dynamic "CloseConnection.vi"("Communicator in"=w123) -> ("error out"=w122:errorcluster)  [unwired: 9 in, 1 out]
            n129 = call <vilib>:"Clear Errors.vi"("error in (no error)"=w122) -> ()  [unwired: 5 in, 2 out]
            n130 = Bundle By Name(cluster=w120, "ICL.exe started"=FALSE, "Communicator"=refnum<class "Communicator.lvclass"> refnum) -> (w121:T3)
          }
          event User Event {
            # "Another Module called the \"SendJSONandAskForReply\" API Method."
            n131 = event-data() -> ("JSON to be sent"=w133:string, "Delay between send and receive [ms]"=w131:i32, "Wait Notifier"=w139:refnum<notifier>, "wait for reply"=w138:bool)  [unwired: 1 in]
            n132 = Unbundle By Name(w135) -> ("Communicator"=w134:refnum<class "Communicator.lvclass">)
            n133 = call-dynamic "SendAndAskForReply.vi"("error in (no error)"=w132, "timeout for receiving data [ms]"=w131, "String to be sent"=w133, "Communicator in"=w134) -> ("error out"=w129:errorcluster, "Data"=w130:string)  [unwired: 5 in, 1 out]
            n134 = Bundle By Name(cluster=T6 {"JSON reply"="", "error"={"status"=FALSE, "code"=0, "source"=""}} ("SendJSONandAskForReply (Reply Payload)"), "JSON reply"=w130, "error"=w129) -> (w137:T6)
            n135 = case "DQMH_FIRE_NOTIFIER" shown="True" w138 {
              tunnel: w139 -> [_ w142]
              tunnel: w137 -> [_ w141]
              frame False {
              }
              frame True {
                n136 = Send Notification(notification=w141, notifier=w142) -> ()  [unwired: 1 in, 2 out]
              }
            }
          }
          event User Event {
            w146 = u32 5000 ("timeout for receiving data [ms]")
            # "#Todo: change timeout from constant to control"
            # "Another Module called the \"DiscoverDevices\" API Method."
            n137 = event-data() -> ("Wait Notifier"=w158:refnum<notifier>, "wait for reply"=w157:bool)  [unwired: 1 in]
            n138 = Unbundle By Name(w155) -> ("Communicator"=w148:refnum<class "Communicator.lvclass">)
            n139 = call "AskForConnectedMonos.vi"("DiscoverDevices in"=T7 {"Monos"=[], "CCDs"=[], "SCDs"=[], "error"={"status"=FALSE, "code"=0, "source"=""}}, "error in (no error)"=w144, "timeout for receiving data [ms]"=w146, "Communicator in"=w148) -> ("error out"=w143:errorcluster, "DiscoverDevices out"=w145:T7, "Communicator out"=w147:refnum<class "Communicator.lvclass">)  [unwired: 5 in]
            n140 = call "AskForConnectedCCDs.vi"("DiscoverDevices in"=w145, "error in (no error)"=w143, "timeout for receiving data [ms]"=w146, "Communicator in"=w147) -> ("error out"=w152:errorcluster, "DiscoverDevices out"=w153:T7, "Communicator out"=w154:refnum<class "Communicator.lvclass">)  [unwired: 5 in]
            n141 = call "AskForConnectedSCDs.vi"("DiscoverDevices in"=w153, "error in (no error)"=w152, "timeout for receiving data [ms]"=w146, "Communicator in"=w154) -> ("error out"=w151:errorcluster, "DiscoverDevices out"=w150:T7)  [unwired: 5 in, 1 out]
            n142 = Bundle By Name(cluster=w150, "error"=w151) -> (w156:T7)
            n143 = case "DQMH_FIRE_NOTIFIER" shown="True" w157 {
              tunnel: w158 -> [_ w161]
              tunnel: w156 -> [_ w160]
              frame False {
              }
              frame True {
                n144 = Send Notification(notification=w160, notifier=w161) -> ()  [unwired: 1 in, 2 out]
              }
            }
          }
        }
        n145 = call-dynamic "Delacor_lib_QMH_Error Handler - Helper Loop.vi"("Error Debug"=w67, "error in"=w69, "Message Queue in"=w68) -> ("dup error in"=w64:errorcluster)  [unwired: 7 in, 1 out]
      }
      n146 = Unregister For Events(event registration refnum=w53) -> ()  [unwired: 1 in, 1 out]
      n147 = Unregister For Events(event registration refnum=w43) -> ()  [unwired: 1 in, 1 out]
    }
    frame Error {
      # "Synchronize Caller Events.vi will inform Start Module.vi that the module has launched and will let the code calling Start Module.vi register for broadcasts and would permit the caller receive the broadcast that an error occurred at launch time."
      n148 = call-dynamic "Delacor_lib_QMH_Release Message Queue.vi"("error in"=w370, "Message Queue"=w363) -> ("error out"=w369:errorcluster)  [unwired: 9 in]
      n149 = call "Synchronize Caller Events.vi"("Singleton Module Admin in"=w364) -> ("error out"=w371:errorcluster)  [unwired: 9 in, 1 out]
      n150 = call "Module Name--constant.vi"() -> ("Module Name"=w367:string)  [unwired: 11 in]
      n151 = Format Into String(format string="An error occurred during initialization. %s is no longer running.", w367) -> (resulting string=w365:string)  [unwired: 2 in, 1 out]
      n152 = Merge Errors(w369, w371) -> (w372:errorcluster)
      n153 = call "Error Reported.vi"("Additional Information"=w365, "Error"=w372) -> ()  [unwired: 9 in, 1 out]
    }
  }
  n154 = Merge Errors(w35, w38) -> (w34:errorcluster)
  n155 = call <vilib>:"Clear Errors.vi"("error in (no error)"=w11) -> ("error out"=w7:errorcluster)  [unwired: 5 in, 1 out]
  n156 = call "Close Module.vi"("error in"=w34, "Module Admin in"=w29) -> ("error out"=w36:errorcluster, "External Launch"=w23:bool, "Module Admin out"=w24:refnum<class "Delacor_lib_QMH_Module Admin.lvclass">)  [unwired: 7 in]
  n157 = call-dynamic "stdin.write.vi"("error in (no error)"=w7, "stdin"="exit", "dotnet_system_exec in"=w12) -> ("error out"=w13:errorcluster, "dotnet_system_exec out"=w10:refnum<class "dotnet_system_exec.lvclass">)  [unwired: 7 in]
  n158 = call "Stall Data Flow.vim"("value in"=w13, "milliseconds to wait"=u32 2000) -> ("value out"=w2:errorcluster)  [unwired: 1 out]
  n159 = Unregister For Events(event registration refnum=w28, error in=w36) -> (error out=w33:errorcluster)
  n160 = call-dynamic "@destroy.vi"("error in (no error)"=w2, "dotnet_system_exec in"=w10) -> ("error out"=w8:errorcluster)  [unwired: 8 in, 1 out]
  n161 = case "External Launch?" shown="True" w23 {
    tunnel: w33 -> [_ w373]
    frame False {
    }
    frame True {
      n162 = case shown="No Error" w373 {
        frame No Error {
          n163 = invoke class="VI" method="FP.Close"() -> ()  [unwired: 3 in, 3 out]
        }
        frame Error {
          n164 = invoke class="VI" method="FP.Open"("Activate"=TRUE ("Activate?")) -> ()  [unwired: 4 in, 5 out]
        }
      }
    }
  }
  n165 = local write "Module Admin"(w24) -> ()
  n166 = Merge Errors(w33, w8) -> (→"error out":errorcluster)
